vi "set cluster.vi"(5 "Value":variant, 7 "Label":string, 8 "error in (no error)":errorcluster, 10 "Layer arrary":string[](array[string])=["Cluster", "Cluster 2", "Cluster 3"], 11 "cluster ref":refnum<vi>) -> (0 "error out":errorcluster, 2 "Acknowledge message":string)   [LabVIEW 2020, in "ui-testing.lvlib"]
uses:
  ui-testing.lvlib
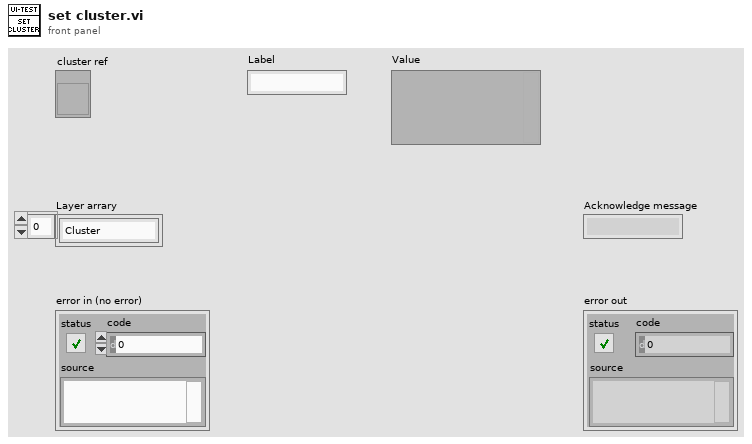
[diagram p1: front panel]
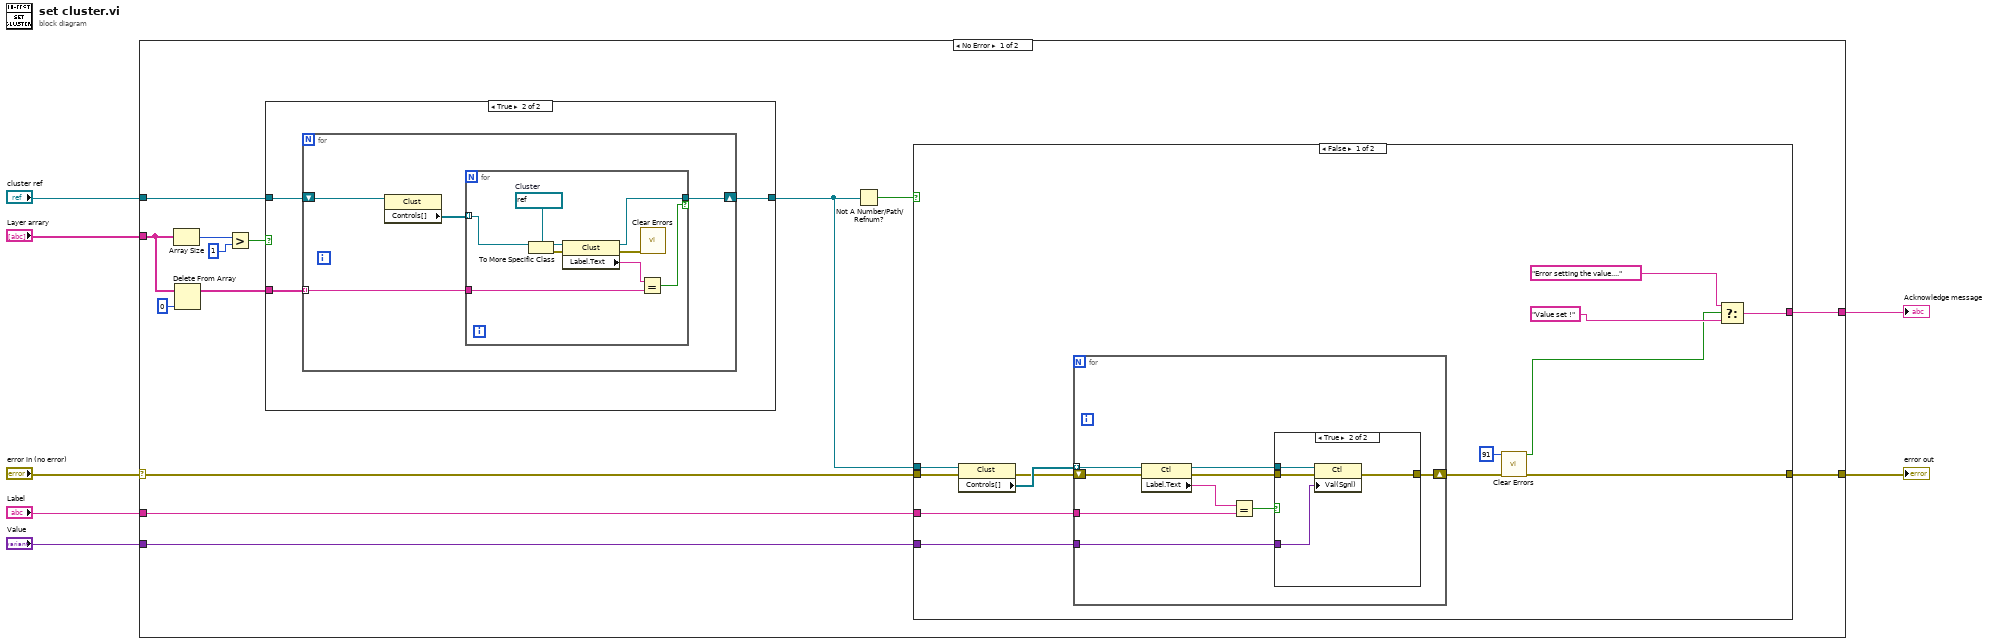
[diagram p0: block diagram]
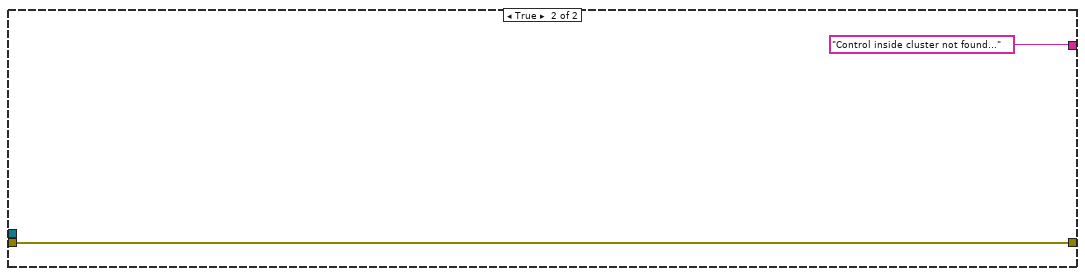
[diagram p3: hidden frame]
diagram:
  n1 = case shown="No Error" "error in (no error)" {
    selector: "error in (no error)" -> [w12 w68]
    tunnel: "Layer arrary" -> [w19 _]
    tunnel: "Label" -> [w15 _]
    tunnel: "cluster ref" -> [w14 _]
    tunnel: "Value" -> [w13 _]
    tunnel: [w11 w68] -> w2
    tunnel: [w10 _] -> w1
    frame No Error {
      n2 = Array Size(array=w19) -> (size(s)=w18:i32)
      n3 = Delete From Array(array=w19, index=0) -> (array with subset deleted=w20:string[])  [unwired: 1 in, 1 out]
      n4 = Greater?(x=w18, y=1) -> (0:w16:bool)
      n5 = case shown="True" w16 {
        tunnel: w14 -> [w51 w54]
        tunnel: w20 -> [_ w53]
        tunnel: [w51 w52] -> w9
        frame False {
        }
        frame True {
          n6 = for {
            tunnel: w53 -> [w56] mode=indexing
            shift-right: [w55] -> w52
            shift-left: w54 -> [w58]
            n7 = property class="Clust"(reference=w58) -> ("Controls[]"=w57:refnum<vi>[])  [unwired: 1 in, 2 out]
            n8 = for {
              tunnel: w57 -> [w67] mode=indexing
              tunnel: w56 -> [w63]
              tunnel: [w61] -> w55 if=w60
              w66 = refnum<vi> refnum  # Cluster
              n9 = To More Specific Class(target class=w66, reference=w67) -> (specific class reference=w65:refnum<vi>, error out=w64:errorcluster)  [unwired: 1 in]
              n10 = property class="Clust"(reference=w65, error in=w64) -> (reference out=w61:refnum<vi>, error out=w59:errorcluster, "Label.Text"=w62:string)
              n11 = Equal?(x=w62, y=w63) -> (x = y?=w60:bool)
              n12 = call <vilib>:"Clear Errors.vi"("error in (no error)"=w59) -> ()  [unwired: 5 in, 2 out]
            }
          }
        }
      }
      n13 = Not A Number/Path/Refnum?(number/path/refnum=w9) -> (NaN/Path/Refnum?=w8:bool)
      n14 = case shown="False" w8 {
        tunnel: w15 -> [w34 _]
        tunnel: w13 -> [w33 _]
        tunnel: w12 -> [w31 w49]
        tunnel: [w28 w49] -> w11
        tunnel: [w23 "Control inside cluster not found..."] -> w10
        tunnel: w9 -> [w22 _]
        frame False {
          n15 = property class="Clust"(reference=w22, error in=w31) -> (error out=w30:errorcluster, "Controls[]"=w32:refnum<vi>[])  [unwired: 1 out]
          n16 = for {
            tunnel: w34 -> [w43]
            tunnel: w32 -> [w41] mode=indexing
            tunnel: w33 -> [w37]
            shift-right: [w35] -> w29
            shift-left: w30 -> [w36]
            n17 = property class="Ctl"(reference=w41, error in=w36) -> (reference out=w39:refnum<vi>, error out=w38:errorcluster, "Label.Text"=w42:string)
            n18 = Equal?(x=w42, y=w43) -> (x = y?=w40:bool)
            n19 = case shown="True" w40 {
              tunnel: w39 -> [_ w48]
              tunnel: w38 -> [w44 w47]
              tunnel: w37 -> [_ w46]
              tunnel: [w44 w45] -> w35
              frame False {
              }
              frame True {
                n20 = property class="Ctl"(reference=w48, error in=w47, "Val(Sgnl)"=w46) -> (error out=w45:errorcluster)  [unwired: 1 out]
              }
            }
          }
          n21 = call <vilib>:"Clear Errors.vi"("error in (no error)"=w29, "specific error code to clear (0: all)"=91) -> ("error out"=w28:errorcluster, "specific error cleared?"=w24:bool)  [unwired: 4 in]
          n22 = Select(t="Error setting the value....", s=w24, f="Value set !") -> (s? t:f=w23:string)
        }
        frame True {
        }
      }
    }
    frame Error {
    }
  }
  "error out" <- w2
  "Acknowledge message" <- w1
